vi "Constructor.vi"(4 "Location":string, 5 "TimeZoneInfoId":string, 6 "OperationCycleStatus":T1=enum."NOT_COMPLETED", 7 "OperationCycleStartTime":timestamp, 8 "error in":errorcluster, 9 "OperationName":string, 10 "ProcessFullName":string, 11 "Name":string) -> (0 "error out":errorcluster, 3 "OperationCycle out":refnum<class "OperationCycle.lvclass">)   [LabVIEW 2021, in "ProligentXMLGenerator.lvlib" / "OperationCycle.lvclass"]
doc: "Defines the operation cycle, which maps the high-level movement (MES level) of a unit within a manufacturing process. \nIt is used to provide more up-to-date information on WIP.\nOperation Cycles are globaly unique by their OperationCycleId property."
uses:
  OperationCycle.lvclass
  OperationCycle.lvclass/OperationCycle.ctl
  Base/DateTime/DateTime.lvclass
  Base/ProcessFullName/ProcessFullName.lvclass
  Base/NonEmptyString_65/NonEmptyString_65.lvclass
  Base/ExecutionStatus/ExecutionStatus.lvclass
  Data.ctl
  Base/NonEmptyString_255/NonEmptyString_255.lvclass
  Base/FullName/FullName.lvclass
  Base/Guid/Guid.lvclass
  Base/NonEmptyString_64/NonEmptyString_64.lvclass
  Model/CustomData/CustomData.lvclass
  Base/ExecutionStatus/Value.ctl
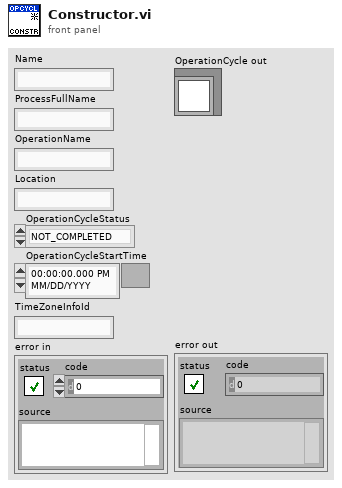
[diagram p1: front panel]
types:
  T1 = typedef "ProligentXMLGenerator.lvlib/ExecutionStatus.lvclass/Value.ctl" = enum16{"PASS", "FAIL", "NOT_COMPLETED", "ABORTED"}
  T2 = typedef "ProligentXMLGenerator.lvlib/OperationCycle.lvclass/Data.ctl" = cluster{"Name":string, "CustomData":refnum<class "CustomData.lvclass">, "ProcessFullName":refnum<class "ProcessFullName.lvclass">, "ProcessVersion":refnum<class "NonEmptyString_64.lvclass">, "OperationCycleId":refnum<class "Guid.lvclass">, "OperationName":refnum<class "NonEmptyString_65.lvclass">, "Location":refnum<class "FullName.lvclass">, "User":refnum<class "NonEmptyString_255.lvclass">, "OperationCycleStatus":refnum<class "ExecutionStatus.lvclass">, "OperationCycleStartTime":refnum<class "DateTime.lvclass">, "OperationCycleEndTime":refnum<class "DateTime.lvclass">, "TimeZoneInfoId":string}
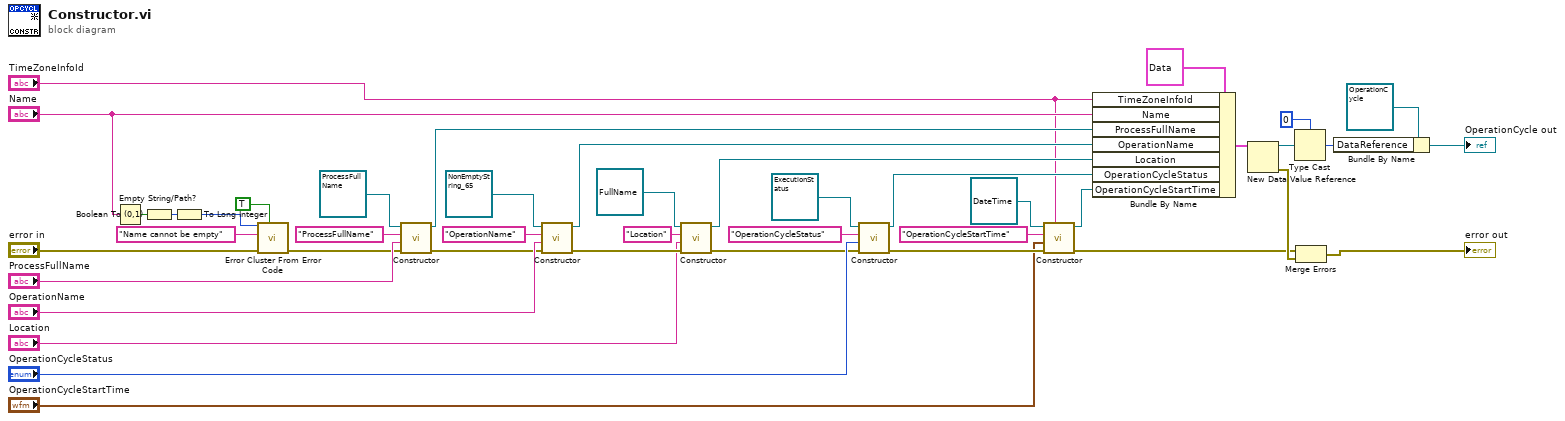
[diagram p0: block diagram]
diagram:
  n1 = Empty String/Path?(string/path="Name") -> (empty?=w27:bool)
  n2 = Boolean To (0,1)(Boolean=w27) -> (0, 1=w26:i16)
  n3 = To Long Integer(number=w26) -> (32bit integer=w25:i32)
  n4 = call <vilib>:"Error Cluster From Error Code.vi"("show call chain? (False)"=TRUE, "error in (no error)"="error in", "error message (\"\")"="Name cannot be empty" ("error message (\"\")"), "error code (0)"=w25) -> ("error out"=w21:errorcluster)  [unwired: 5 in]
  n5 = call-dynamic "Constructor.vi"("error in"=w21, "Value"="ProcessFullName", "Name"="ProcessFullName", "String in"=refnum<class "ProcessFullName.lvclass"> refnum ("ProligentResultProcessor:ProcessFullName")) -> ("error out"=w16:errorcluster, "String out"=w22:refnum<class "ProcessFullName.lvclass">)  [unwired: 6 in]
  n6 = call-dynamic "Constructor.vi"("error in"=w16, "Value"="OperationName", "Name"="OperationName", "String in"=refnum<class "NonEmptyString_65.lvclass"> refnum ("ProligentResultProcessor:NonEmptyString_65")) -> ("error out"=w7:errorcluster, "String out"=w15:refnum<class "NonEmptyString_65.lvclass">)  [unwired: 6 in]
  n7 = call-dynamic "Constructor.vi"("error in"=w7, "Value"="Location", "Name"="Location", "String in"=refnum<class "FullName.lvclass"> refnum ("ProligentResultProcessor:FullName")) -> ("error out"=w6:errorcluster, "String out"=w4:refnum<class "FullName.lvclass">)  [unwired: 6 in]
  n8 = call-dynamic "Constructor.vi"("error in"=w6, "Value"="OperationCycleStatus", "Name"="OperationCycleStatus", "ExecutionStatus in"=refnum<class "ExecutionStatus.lvclass"> refnum ("ProligentResultProcessor:ExecutionStatus")) -> ("error out"=w13:errorcluster, "ExecutionStatus out"=w10:refnum<class "ExecutionStatus.lvclass">)  [unwired: 6 in]
  n9 = call-dynamic "Constructor.vi"("TimeZoneInfoId"="TimeZoneInfoId", "error in"=w13, "Value"="OperationCycleStartTime", "Name"="OperationCycleStartTime", "DateTime in"=refnum<class "DateTime.lvclass"> refnum) -> ("error out"=w20:errorcluster, "DateTime out"=w29:refnum<class "DateTime.lvclass">)  [unwired: 5 in]
  n10 = Bundle By Name(cluster=T2 {"Name"="", "CustomData"=refnum, "ProcessFullName"=refnum, "ProcessVersion"=refnum, "OperationCycleId"=refnum, "OperationName"=refnum, "Location"=refnum, "User"=refnum, "OperationCycleStatus"=refnum, "OperationCycleStartTime"=refnum, "OperationCycleEndTime"=refnum, "TimeZoneInfoId"=""} ("Data"), "TimeZoneInfoId"="TimeZoneInfoId", "Name"="Name", "ProcessFullName"=w22, "OperationName"=w15, "Location"=w4, "OperationCycleStatus"=w10, "OperationCycleStartTime"=w29) -> (w34:T2)
  n11 = New Data Value Reference(data value=w34) -> (data value reference=w33:refnum<data-value>, error out=w30:errorcluster)  [unwired: 1 in]
  n12 = Type Cast(type=u64 0, x=w33) -> (*(type *) &x=w31:u64)
  n13 = Merge Errors(w20, w30) -> (→"error out":errorcluster)
  n14 = Bundle By Name(cluster=refnum<class "OperationCycle.lvclass"> refnum ("ProligentResultProcessor:OperationRun"), "DataReference"=w31) -> (→"OperationCycle out":refnum<class "OperationCycle.lvclass">)
